vi "Set Point.vi"(8 "error in (no error)":errorcluster, 10 "Set point":dbl, 11 "Cryo-Con Driver in":refnum<class "Cryo-Con Driver.lvclass">) -> (0 "error out":errorcluster, 3 "Cryo-Con Driver out":refnum<class "Cryo-Con Driver.lvclass">)   [LabVIEW 2016, in "Cryo-Con Driver.lvclass"]
uses:
  Cryo-Con Driver.lvclass
  C:/github/NHMFL_Core/Libraries/Instruments/VISA Instrument/VISA Instrument.lvclass
  VISA Instrument/VISA Instrument.lvclass/VISA Instrument.ctl
  VISA Instrument/Read VISA resource.vi
  VISA Instrument/Write VISA resource.vi
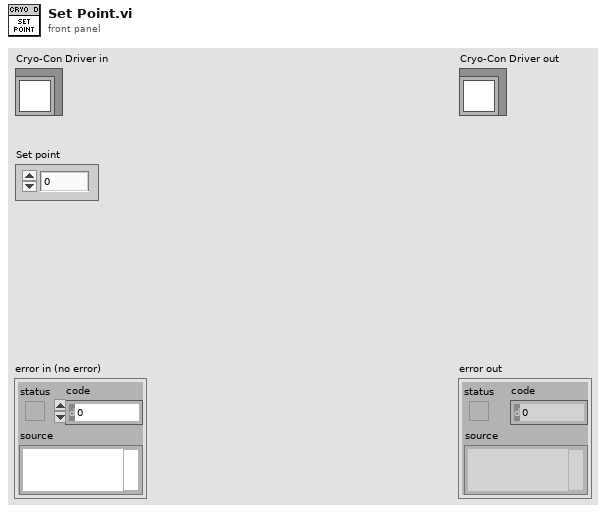
[diagram p1: front panel]
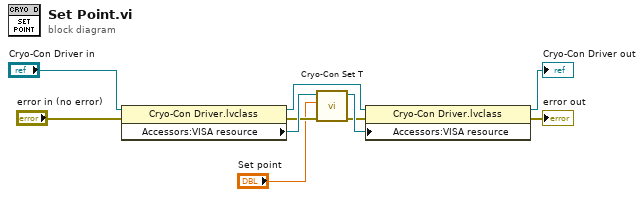
[diagram p0: block diagram]
diagram:
  n1 = property class="Cryo-Con Driver.lvclass"(reference="Cryo-Con Driver in", error in="error in (no error)") -> (reference out=w10:refnum<class "Cryo-Con Driver.lvclass">, error out=w5:errorcluster, "Accessors:VISA resource"=w8:refnum<visa-resource-name>)
  n2 = call "Cryo-Con Set T.vi"("error in (no error)"=w5, "Set T"="Set point", "VISA Resource Name"=w8) -> ("error out"=w6:errorcluster, "VISA Resource Name Out"=w7:refnum<visa-resource-name>)  [unwired: 7 in]
  n3 = property class="Cryo-Con Driver.lvclass"(reference=w10, error in=w6, "Accessors:VISA resource"=w7) -> (reference out=→"Cryo-Con Driver out":refnum<class "Cryo-Con Driver.lvclass">, error out=→"error out":errorcluster)
